vi "Agilent VNA Preset.vi"(7 "Agilent VNA":T1, 8 "error in (no error)":errorcluster, 11 "VISA Resource Name":refnum<visa-resource-name>) -> (0 "error out":errorcluster, 3 "dup VISA Resource Name":refnum<visa-resource-name>)   [LabVIEW 2011]
uses:
  TypeDefs/Agilent VNA Instrument Info.ctl
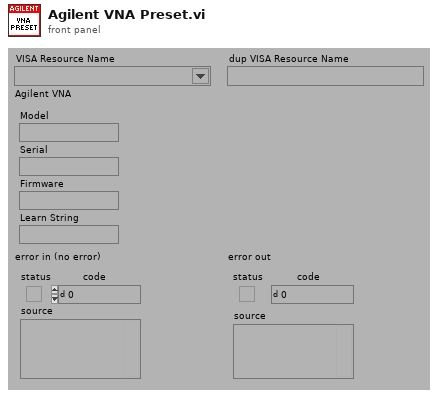
[diagram p1: front panel]
types:
  T1 = typedef "Agilent VNA Instrument Info.ctl" = cluster{"Model":string, "Serial":string, "Firmware":string, "Learn String":string}
  T2 = typedef "Agilent VNA Model.ctl" = enum16{"Not Supported", "8510X", "8719X", "8720X", "8722X", "8753X", "ENA", "PNA", "Field Fox"}
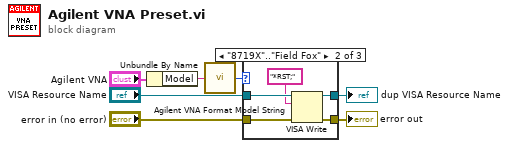
[diagram p0: block diagram]
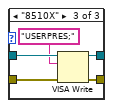
[diagram p3: hidden frame]
diagram:
  n1 = Unbundle By Name("Agilent VNA") -> ("Model"=w1:string)
  n2 = call "Agilent VNA Format Model String.vi"("Model"=w1) -> ("Model"=w3:T2)
  n3 = case shown="\"8719X\"..\"Field Fox\"" w3 {
    tunnel: "error in (no error)" -> [w8 w14 w19]
    tunnel: "VISA Resource Name" -> [w9 w13 w18]
    tunnel: [w9 w12 w17] -> w5
    tunnel: [w8 w11 w16] -> w4
    frame "Not Supported" {
    }
    frame "8719X".."Field Fox" {
      n4 = VISA Write(VISA resource name=w13, write buffer="*RST;", error in (no error)=w14) -> (VISA resource name out=w12:refnum<visa-resource-name>, error out=w11:errorcluster)  [unwired: 1 out]
    }
    frame "8510X" {
      n5 = VISA Write(VISA resource name=w18, write buffer="USERPRES;", error in (no error)=w19) -> (VISA resource name out=w17:refnum<visa-resource-name>, error out=w16:errorcluster)  [unwired: 1 out]
    }
  }
  "error out" <- w4
  "dup VISA Resource Name" <- w5
